vi "T1.vi"() -> ()   [LabVIEW 2020]
panel:
  out "Restul Impartirii":dbl
  out "Catul Impartirii":dbl
  in  "B":dbl
  in  "A":dbl
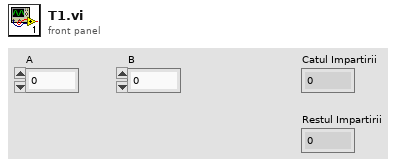
[diagram p1: front panel]
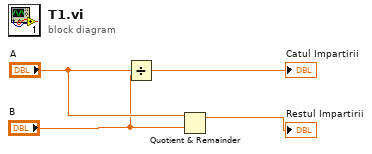
[diagram p0: block diagram]
diagram:
  n1 = Divide(x="A", y="B") -> (x/y=→"Catul Impartirii":dbl)
  n2 = Quotient & Remainder(x="A", y="B") -> (x-y*floor(x/y)=→"Restul Impartirii":dbl)  [unwired: 1 out]
